vi "create.vi"(8 "error in (no error)":errorcluster) -> (0 "error out":errorcluster, 3 "system.threading out":refnum<class "system.threading.lvclass">)   [LabVIEW 2021, in "system.threading.lvclass"]
uses:
  system.threading.lvclass
  system.threading.lvclass/system.threading.ctl
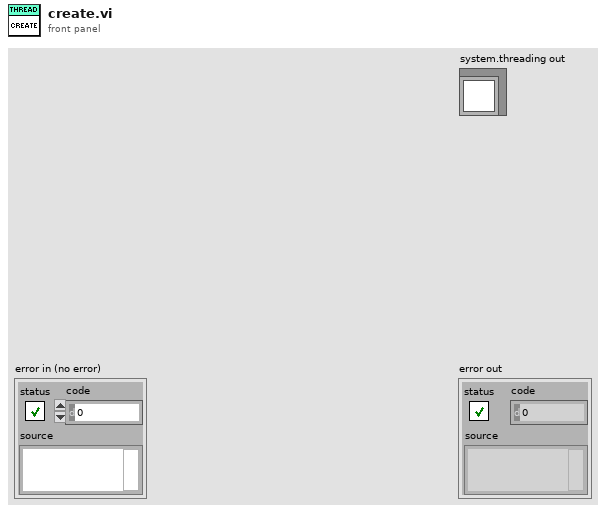
[diagram p1: front panel]
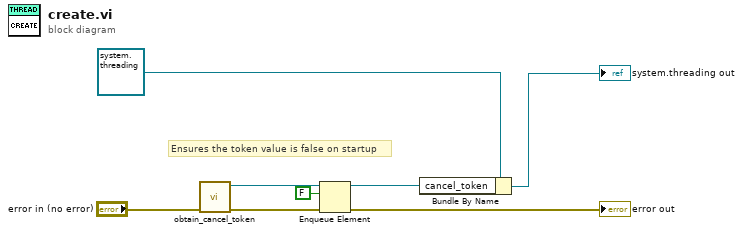
[diagram p0: block diagram]
diagram:
  # "Ensures the token value is false on startup"
  n1 = call "obtain_cancel_token.vi"("error in (no error)"="error in (no error)") -> ("error out"=w5:errorcluster, "cancel_token"=w4:refnum<queue>)  [unwired: 9 in]
  n2 = Enqueue Element(queue=w4, element=FALSE, error in (no error)=w5) -> (queue out=w2:refnum<queue>, error out=→"error out":errorcluster)  [unwired: 1 in, 1 out]
  n3 = Bundle By Name(cluster=refnum<class "system.threading.lvclass"> refnum ("system.threading in"), "cancel_token"=w2) -> (→"system.threading out":refnum<class "system.threading.lvclass">)
